vi "Main.vi"() -> ()   [LabVIEW 2024]
uses:
  Data Generator API/Data Generator API.lvclass
  C:/Users/320141162/Desktop/DUTLug3/API/API.lvclass
  API/API.lvclass
  Data Generator Actor/Data Generator Actor.lvclass
panel:
  in  "Actor Selector":bool
  in  "New Count":i32
  out "current time":timestamp
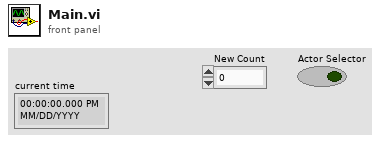
[diagram p1: front panel]
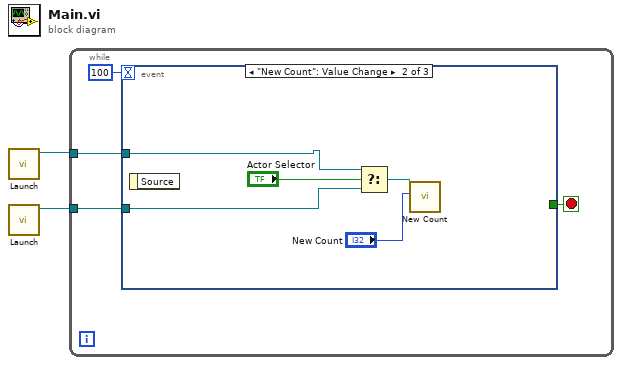
[diagram p0: block diagram]
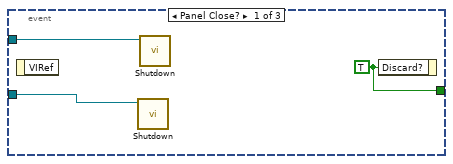
[diagram p2: hidden frame]
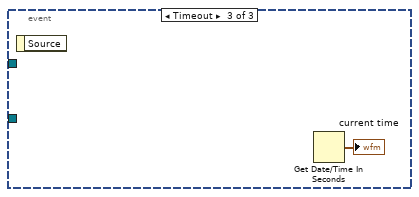
[diagram p3: hidden frame]
diagram:
  n1 = call "Launch.vi"() -> ("Data Generator API.lvclass"=w2:refnum<class "Data Generator API.lvclass">)  [unwired: 11 in]
  n2 = call "Launch.vi"() -> ("Data Generator API.lvclass"=w1:refnum<class "Data Generator API.lvclass">)  [unwired: 11 in]
  n3 = while {
    tunnel: w2 -> [w4]
    tunnel: w1 -> [w3]
    stop <- w5 stop-if-true
    n4 = event shown="[1] \"New Count\": Value Change" {
      selector: _ -> [_ _ _]
      dyn-events: _ -> [_ _ _]
      timeout: 100 -> [_ _ _]
      tunnel: [w9 _ _] -> w5
      tunnel: w4 -> [w8 w14 _]
      tunnel: w3 -> [w7 w13 _]
      event Panel Close? {
        w9 = TRUE ("Discard?")
        n5 = event-data() -> ()  [unwired: 1 in, 1 out]
        n6 = call "Shutdown.vi"("API in"=w7) -> ()  [unwired: 11 in]
        n7 = call "Shutdown.vi"("API in"=w8) -> ()  [unwired: 11 in]
        n8 = event-data("Discard?"=w9) -> ()  [unwired: 1 in, 1 out]
      }
      event "New Count": Value Change {
        n9 = event-data() -> ()  [unwired: 1 in, 1 out]
        n10 = Select(t=w14, s="Actor Selector", f=w13) -> (s? t:f=w12:refnum<class "Data Generator API.lvclass">)
        n11 = call "New Count.vi"("New Count"="New Count", "API in"=w12) -> ()  [unwired: 10 in]
      }
      event Timeout {
        n12 = event-data() -> ()  [unwired: 1 in, 1 out]
        n13 = Get Date/Time In Seconds() -> (seconds since 1Jan1904=→"current time":timestamp)
      }
    }
  }
